vi "Read Timing Source.vi"(8 "Error In":errorcluster caption="error in", 11 "Custom Device .NET Ref In":refnum<k24>) -> (0 "Error Out":errorcluster caption="error in", 2 "Timing Source Properties":T1, 3 "Custom Device .NET Ref Out":refnum<k24>)   [LabVIEW 2015, in "VeriStand XML Parser.lvlib"]
doc: "Reads and returns the timing source properties of the custom device"
uses:
  VeriStand XML Parser.lvlib
  NationalInstruments.VeriStand.XMLReader
  XML Controls/Timing Source Properties.ctl
  XML Controls/Timing Source Source Distribution Properties.ctl
  XML Controls/Supported Targets.ctl
  XML Controls/Path Cluster.ctl
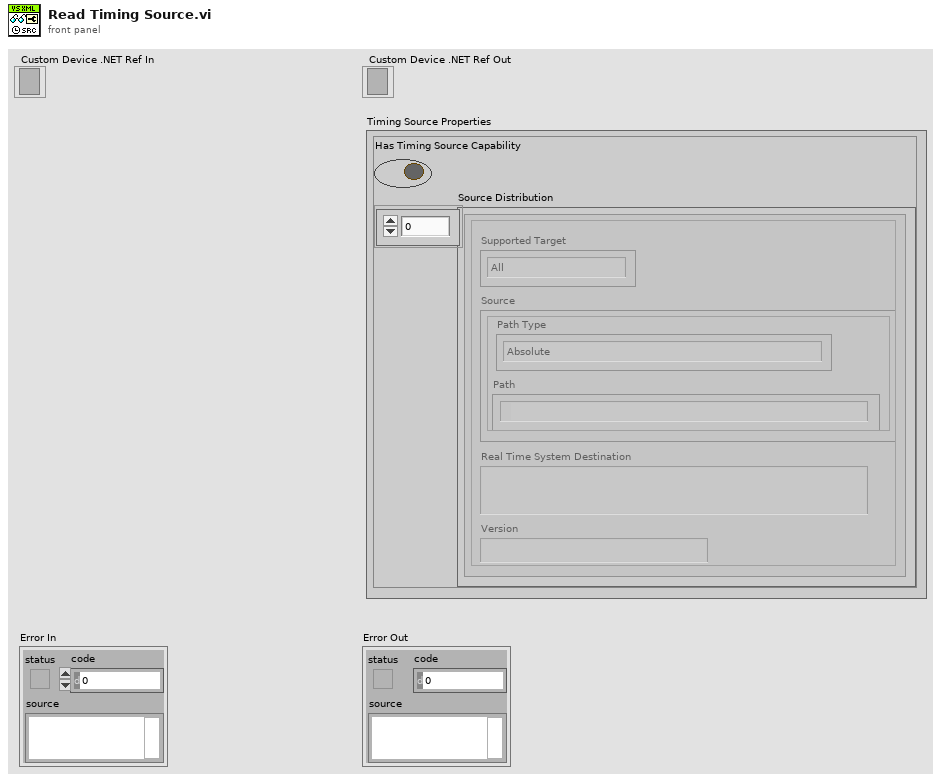
[diagram p1: front panel]
types:
  T1 = typedef "VeriStand XML Parser.lvlib/Timing Source Properties.ctl" = cluster{"Has Timing Source Capability":bool, "Source Distribution":T2}
  T2 = typedef "VeriStand XML Parser.lvlib/Timing Source Source Distribution Properties.ctl" = cluster{"Supported Target":T3, "Source":T4, "Real Time System Destination":string, "Version":string}[]
  T3 = typedef "VeriStand XML Parser.lvlib/Supported Targets.ctl" = enum16{"All", "Pharlap", "VxWorks", "Windows", "Linux_32_ARM", "Linux_x64", "PharlapWindows", "PharlapVxWorks", "VxWorksWindows"}
  T4 = typedef "VeriStand XML Parser.lvlib/Path Cluster.ctl" = cluster{"Path":path, "Path Type":enum16{"Absolute", "To Base", "To Common Doc Dir", "To Application Data Dir"}}
  T5 = cluster{"Supported Target":T3, "Source":T4, "Real Time System Destination":string, "Version":string}
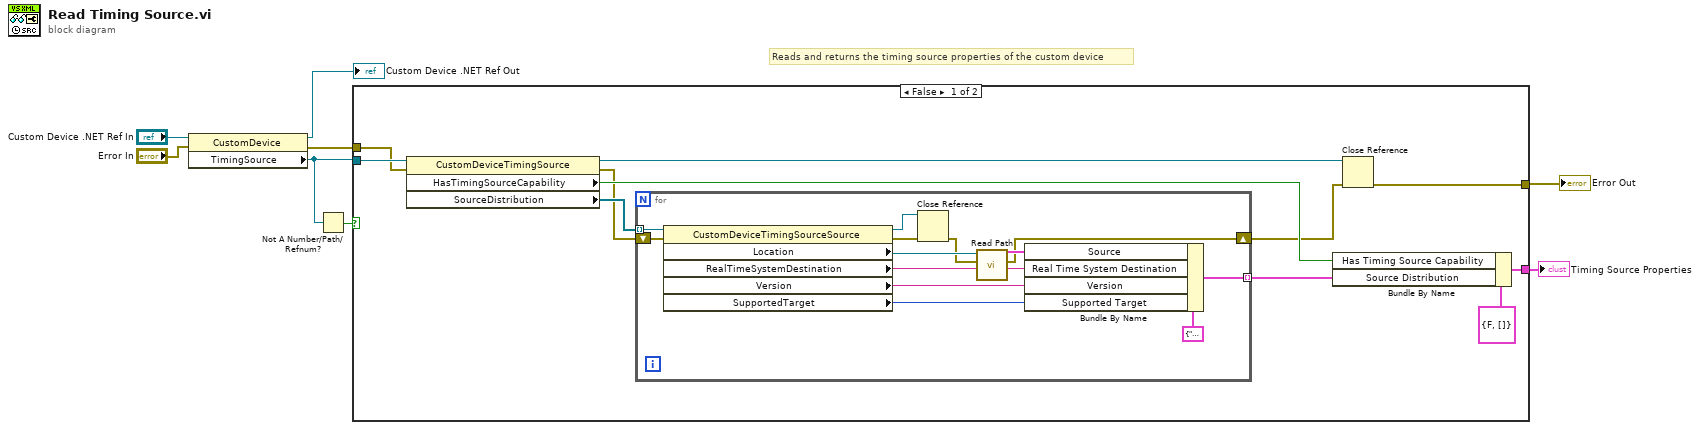
[diagram p0: block diagram]
diagram:
  # "Reads and returns the timing source properties of the custom device"
  n1 = property class="CustomDevice"(reference="Custom Device .NET Ref In", error in="Error In") -> (reference out=→"Custom Device .NET Ref Out":refnum<k24>, error out=w4:errorcluster, "TimingSource"=w3:refnum<k24>)
  n2 = Not A Number/Path/Refnum?(number/path/refnum=w3) -> (NaN/Path/Refnum?=w2:bool)
  n3 = case shown="False" w2 {
    tunnel: w3 -> [w19 _]
    tunnel: w4 -> [w18 w33]
    tunnel: [w15 _] -> w1
    tunnel: [w11 w33] -> w5
    frame False {
      n4 = property class="CustomDeviceTimingSource"(reference=w19, error in=w18) -> (reference out=w13:refnum<k24>, error out=w14:errorcluster, "HasTimingSourceCapability"=w17:bool, "SourceDistribution"=w16:refnum<k24>[])
      n5 = for {
        tunnel: w16 -> [w32] mode=indexing
        tunnel: [w31] -> w9 mode=indexing
        shift-right: [w20] -> w12
        shift-left: w14 -> [w30]
        n6 = property class="CustomDeviceTimingSourceSource"(reference=w32, error in=w30) -> (reference out=w28:refnum<k24>, error out=w23:errorcluster, "Location"=w29:refnum<k24>, "RealTimeSystemDestination"=w27:string, "Version"=w26:string, "SupportedTarget"=w25:i32)
        n7 = Close Reference(reference=w28, error in (no error)=w23) -> (error out=w22:errorcluster)
        n8 = call "Read Path.vi"("Error In"=w22, "Path .NET Ref"=w29) -> ("Error Out"=w20:errorcluster, "Path Properties"=w24:T4)  [unwired: 8 in]
        n9 = Bundle By Name(cluster=T5 {"Supported Target"=enum."All", "Source"={"Path"=path "", "Path Type"=enum."Absolute"}, "Real Time System Destination"="", "Version"=""} ("Source"), "Source"=w24, "Real Time System Destination"=w27, "Version"=w26, "Supported Target"=w25) -> (w31:T5)
      }
      n10 = Bundle By Name(cluster=T1 {"Has Timing Source Capability"=FALSE, "Source Distribution"=[]} ("Timing Source Properties"), "Has Timing Source Capability"=w17, "Source Distribution"=w9) -> (w15:T1)
      n11 = Close Reference(reference=w13, error in (no error)=w12) -> (error out=w11:errorcluster)
    }
    frame True {
    }
  }
  "Error Out" <- w5
  "Timing Source Properties" <- w1
